vi "Debounce.vi"(1 "Input":bool) -> (0 "Output":bool)   [LabVIEW 2016]
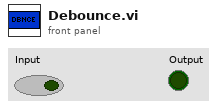
[diagram p1: front panel]
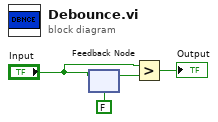
[diagram p0: block diagram]
diagram:
  n1 = feedback #1(FALSE ("Fuel Flap")) -> (w3:bool)
  n2 = feedback-in #1("Input") -> ()
  n3 = Greater?(x="Input", y=w3) -> (0:→"Output":bool)
